vi "Read TDMS (SubVI).vi"(5 "Sensor Y":i32=2, 7 "Sensor X":i32=1, 9 "Rotation":dbl, 10 "i":dbl, 11 "TDMS File Path in":path=path "C:/Users/Clayton/Documents/Mestrado ITA/Dissertacao/Simulacoes Matlab/zLabView/TDMS_teste.tdms") -> (0 "stop":bool, 1 "waveform 3":waveform(dbl), 2 "waveform 2":waveform(dbl), 3 "waveform 1":waveform(dbl))   [LabVIEW 2012]
uses:
  <vilib>/Waveform/WDTOps.llb/WDT Index Channel DBL.vi
  <vilib>/Waveform/WDTOps.llb/WDT Get Waveform Subset DBL.vi
panel:
  out "Rot max":dbl
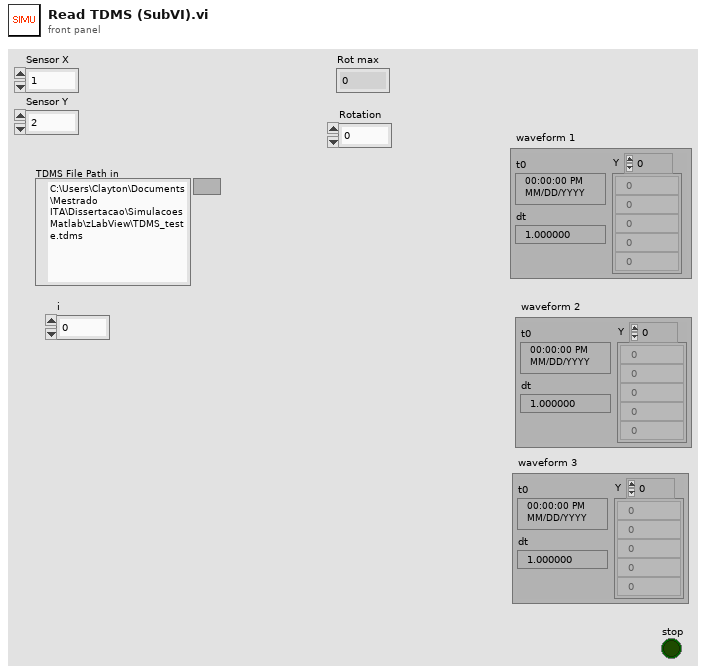
[diagram p1: front panel]
types:
  T1 = enum16{"open", "open or create", "create or replace", "create", "open (read-only)"}
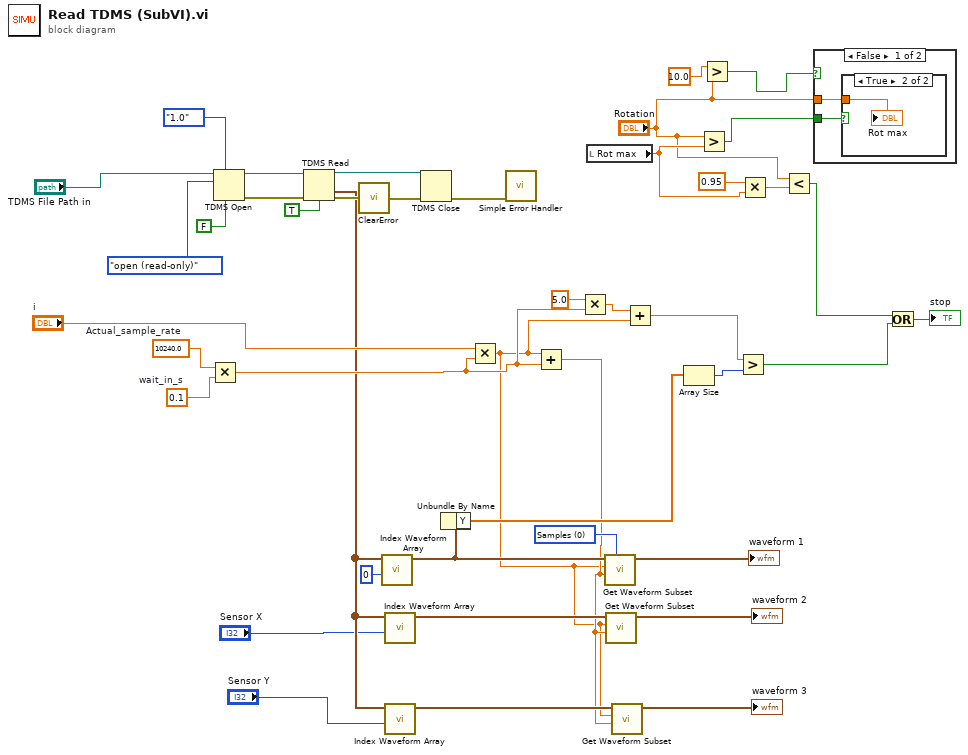
[diagram p0: block diagram]
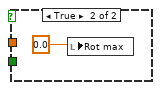
[diagram p3: hidden frame]
diagram:
  w25 = u16 0 items=["Samples", "Relative Time"] ("start/duration format")
  w30 = 0.1  # wait_in_s
  w31 = 10240.0  # Actual_sample_rate
  n1 = Multiply(x=w31, y=w30) -> (x*y=w18:dbl)
  n2 = TDMS Open(6:FALSE ("disable buffering (T)"), 7:enum16{"1.0", "2.0"}."1.0" ("file format version (2.0)"), 10:T1."open (read-only)" ("operation"), 11:"TDMS File Path in") -> (0:w38:errorcluster, 3:w37:refnum<k34>)  [unwired: 2 in]
  n3 = TDMS Read(0:w37, 11:w38, 13:TRUE ("return channels in file order? (F)")) -> (4:w34:refnum<k34>, 10:w13:waveform(dbl)[], 15:w41:errorcluster)  [unwired: 5 in, 3 out]
  n4 = call <vilib>:"ClearError.vi"("error in (no error)"=w41) -> ("error out"=w35:errorcluster)
  n5 = call-poly <vilib>:"Index Waveform Array.vi"("index"=0, "waveform array"=w13) -> ("waveform"=w27:waveform(dbl))  [unwired: 8 in, 1 out]
  n6 = call-poly <vilib>:"Index Waveform Array.vi"("index"="Sensor X", "waveform array"=w13) -> ("waveform"=w22:waveform(dbl))  [unwired: 8 in, 1 out]
  n7 = call-poly <vilib>:"Index Waveform Array.vi"("index"="Sensor Y", "waveform array"=w13) -> ("waveform"=w20:waveform(dbl))  [unwired: 8 in, 1 out]
  n8 = TDMS Close(8:w35, 11:w34) -> (0:w33:errorcluster)  [unwired: 1 out]
  n9 = Unbundle By Name(w27) -> ("Y"=w26:dbl[])
  n10 = Multiply(x="i", y=w18) -> (x*y=w15:dbl)
  n11 = call <vilib>:"Simple Error Handler.vi"("error in (no error)"=w33) -> ()  [unwired: 1 in, 8 out]
  n12 = Add(x=w15, y=w18) -> (x+y=w19:dbl)
  n13 = Multiply(x=5.0, y=w18) -> (x*y=w16:dbl)
  n14 = local read "Rot max"() -> (w4:dbl)
  n15 = call-poly <vilib>:"Get Waveform Subset.vi"("start/duration format"=w25, "duration"=w19, "start samples/time"=w15, "waveform in"=w27) -> ("waveform out"=→"waveform 1":waveform(dbl))  [unwired: 2 in, 3 out]
  n16 = call-poly <vilib>:"Get Waveform Subset.vi"("duration"=w19, "start samples/time"=w15, "waveform in"=w22) -> ("waveform out"=→"waveform 2":waveform(dbl))  [unwired: 3 in, 3 out]
  n17 = call-poly <vilib>:"Get Waveform Subset.vi"("duration"=w19, "start samples/time"=w15, "waveform in"=w20) -> ("waveform out"=→"waveform 3":waveform(dbl))  [unwired: 3 in, 3 out]
  n18 = Add(x=w16, y=w15) -> (x+y=w14:dbl)
  n19 = Array Size(array=w26) -> (size(s)=w28:i32)
  n20 = Greater?(x="Rotation", y=w4) -> (0:w5:bool)
  n21 = Greater?(x=10.0 ("y"), y="Rotation") -> (0:w3:bool)
  n22 = Greater?(x=w14, y=w28) -> (0:w9:bool)
  n23 = Multiply(x=0.95, y=w4) -> (x*y=w6:dbl)
  n24 = Less?(x="Rotation", y=w6) -> (x < y?=w8:bool)
  n25 = case shown="False" w3 {
    tunnel: "Rotation" -> [w45 _]
    tunnel: w5 -> [w44 _]
    frame False {
      n26 = case shown="True" w44 {
        tunnel: w45 -> [_ w46]
        frame False {
        }
        frame True {
          "Rot max" <- w46
        }
      }
    }
    frame True {
      n27 = local write "Rot max"(0.0 ("Rot max")) -> ()
    }
  }
  n28 = Or(x=w8, y=w9) -> (x .or. y?=→"stop":bool)
